vi "Initialize.vi"(8 "error in (no error)":errorcluster, 10 "data":u8[](array[numeric])) -> (0 "error out":errorcluster, 3 "Buffer Upload Controller out":refnum<class "Buffer Upload Controller.lvclass">)   [LabVIEW 2020, in "NI_SFTP.lvlib" / "Buffer Upload Controller.lvclass"]
uses:
  <vilib>/net/SFTP/API/Support/Upload/Buffer/Buffer Upload Controller.lvclass
  <vilib>/net/SFTP/API/Support/Upload/Buffer/Buffer Upload Controller.lvclass/Buffer Upload Controller.ctl
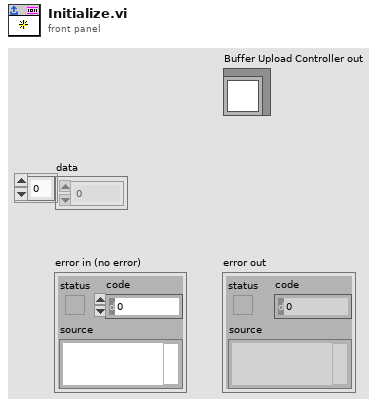
[diagram p1: front panel]
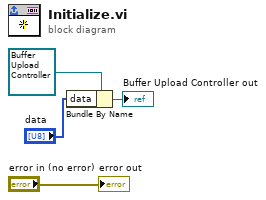
[diagram p0: block diagram]
diagram:
  n1 = Bundle By Name(cluster=refnum<class "Buffer Upload Controller.lvclass"> refnum ("Buffer Upload Controller in"), "data"="data") -> (→"Buffer Upload Controller out":refnum<class "Buffer Upload Controller.lvclass">)
  "error out" <- "error in (no error)"
